vi "initialize Session Data.vi"(0 "Session in":refnum<class "Local Listener Session.lvclass">, 11 "error in":errorcluster) -> (4 "Session out":refnum<class "Local Listener Session.lvclass">, 15 "error out":errorcluster)   [LabVIEW 2012, in "REx.lvlib" / "Local Listener Session.lvclass"]
uses:
  Local Listener Session.lvclass
  <userlib>/_Session Fwk/Session - Root.lvclass
  Local Listener Session.lvclass/Local Listener Session.ctl
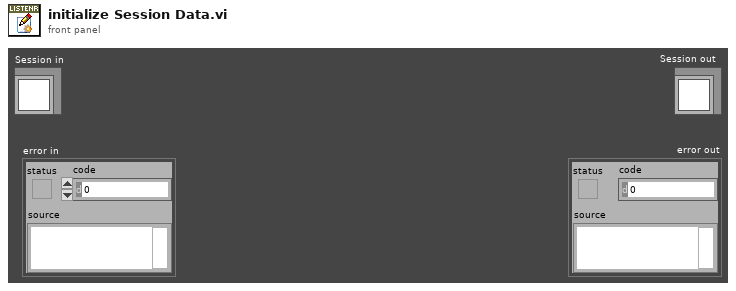
[diagram p1: front panel]
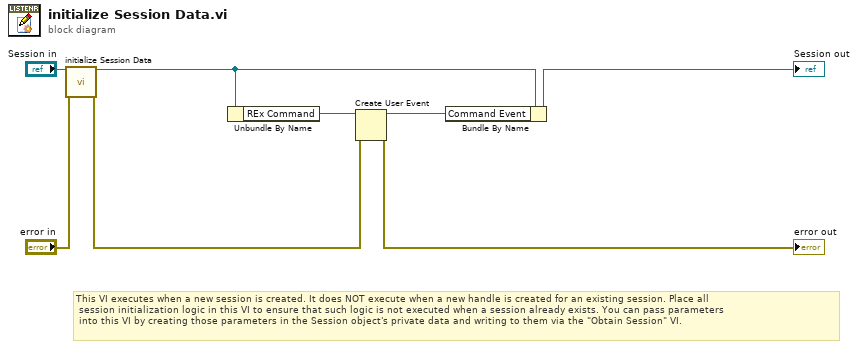
[diagram p0: block diagram]
diagram:
  # "This VI executes when a new session is created. It does NOT execute when a new handle is created for an existing session. Place all\n session initialization logic in this VI to ensure that such logic is not executed when a session already exists. You can pass parameters\n into this VI by creating those parameters in the Session object's private data and writing to them via the \"Obtain Session\" VI."
  n1 = call-parent "initialize Session Data.vi"("OBJ - Session in"="Session in", "error in"="error in") -> ("OBJ - Session out"=w2:refnum<class "Local Listener Session.lvclass">, "error out"=w6:errorcluster)  [unwired: 12 in]
  n2 = Unbundle By Name(w2) -> ("REx Command"=w1:refnum<class "REx Command - Root.lvclass">)
  n3 = Create User Event(user event datatype=w1, error in=w6) -> (user event=w3:refnum<user-event>, error out=→"error out":errorcluster)
  n4 = Bundle By Name(cluster=w2, "Command Event"=w3) -> (→"Session out":refnum<class "Local Listener Session.lvclass">)
